vi "读取产品参数信息-铜片参数.vi"(8 "错误输入（无错误）":errorcluster, 11 "LoadProductName":string) -> (0 "错误输出":errorcluster)   [LabVIEW 2017]
uses:
  Global System.vi
  <vilib>/Utility/xml.llb/Read From XML File(string).vi
panel:
  out "添加的路径":path
  out "连接的字符串":string
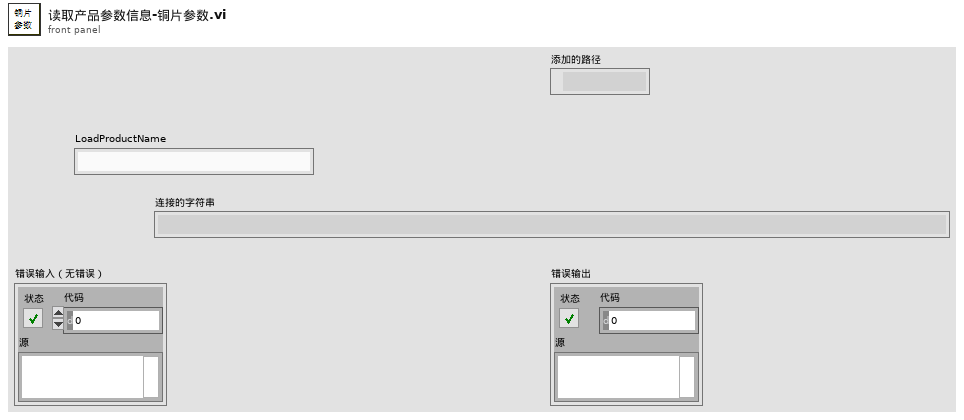
[diagram p1: front panel]
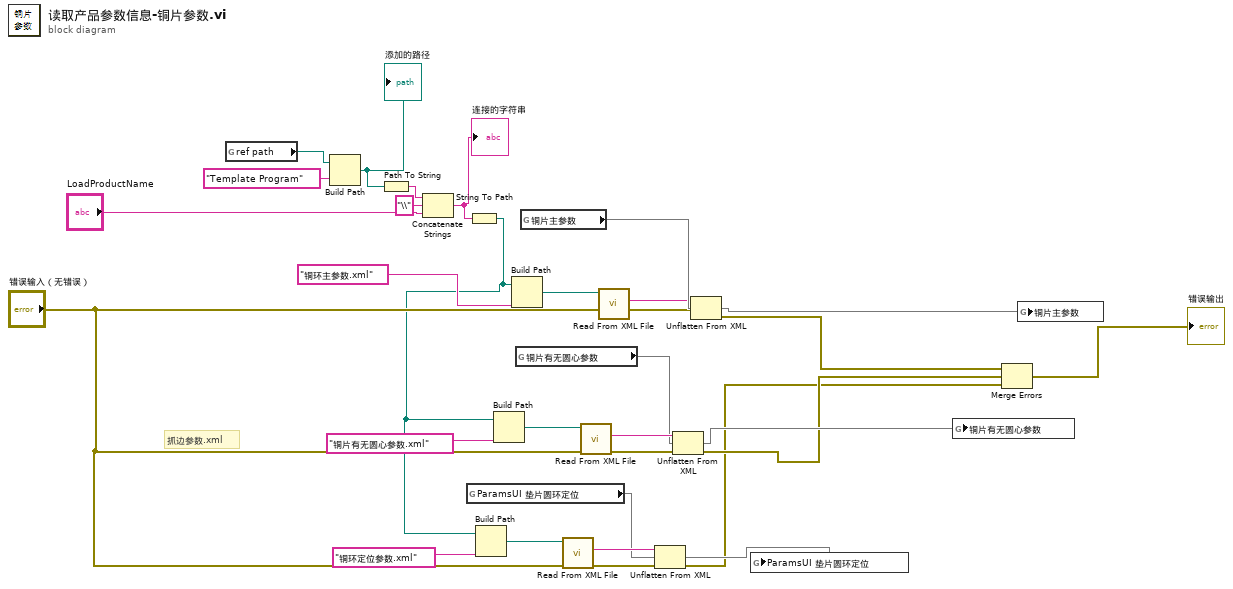
[diagram p0: block diagram]
diagram:
  # "抓边参数.xml"
  n1 = global read "Global System.vi" "ref path"() -> (w28:path)
  n2 = Build Path(base path=w28, name or relative path="Template Program" ("名称或相对路径")) -> (appended path=w26:path)
  "添加的路径" <- w26
  n3 = Path To String(path=w26) -> (string=w25:string)
  n4 = Concatenate Strings(w25, "\\" ("字符串"), "LoadProductName") -> (w22:string)
  "连接的字符串" <- w22
  n5 = global read "Global System.vi" "ParamsUI 垫片圆环定位"() -> (w3)
  n6 = String To Path(string=w22) -> (path=w4:path)
  n7 = Build Path(base path=w4, name or relative path="铜环定位参数.xml" ("名称或相对路径")) -> (appended path=w7:path)
  n8 = Build Path(base path=w4, name or relative path="铜片有无圆心参数.xml" ("名称或相对路径")) -> (appended path=w15:path)
  n9 = Build Path(base path=w4, name or relative path="铜环主参数.xml" ("名称或相对路径")) -> (appended path=w19:path)
  n10 = global read "Global System.vi" "铜片有无圆心参数"() -> (w14)
  n11 = global read "Global System.vi" "铜片主参数"() -> (w21)
  n12 = call-poly <vilib>:"Read From XML File.vi"("XML File Path"=w7) -> ("XML Elements"=w6:string)  [unwired: 8 in, 2 out]
  n13 = call-poly <vilib>:"Read From XML File.vi"("XML File Path"=w15) -> ("XML Elements"=w16:string)  [unwired: 8 in, 2 out]
  n14 = call-poly <vilib>:"Read From XML File.vi"("XML File Path"=w19) -> ("XML Elements"=w18:string)  [unwired: 8 in, 2 out]
  n15 = Unflatten From XML(xml string=w6, type=w3, error in (no error)="错误输入（无错误）") -> (value=w2, error out=w1:errorcluster)
  n16 = Unflatten From XML(xml string=w16, type=w14, error in (no error)="错误输入（无错误）") -> (value=w13, error out=w11:errorcluster)
  n17 = Unflatten From XML(xml string=w18, type=w21, error in (no error)="错误输入（无错误）") -> (value=w17, error out=w12:errorcluster)
  n18 = global write "Global System.vi" "ParamsUI 垫片圆环定位"(w2) -> ()
  n19 = global write "Global System.vi" "铜片有无圆心参数"(w13) -> ()
  n20 = Merge Errors(w12, w11, w1) -> (→"错误输出":errorcluster)
  n21 = global write "Global System.vi" "铜片主参数"(w17) -> ()
